vi "Teleop.vi"(10 "Match Info":T1={"Autonomous Elapsed Seconds"=0.0, "TeleOp Elapsed Seconds"=0.0, "Disabled Elapsed Seconds"=0.0, "Visited Autonomous"=FALSE, "Visited TeleOp"=FALSE, "Visited Disabled"=FALSE, "Autonomous Settings"={"Autonomous Style"=enum."Independent", "VI Refnum"=refnum}}, 11 "Call Context":T2) -> ()   [LabVIEW 2011]
doc: "This VI is called for each TeleOp packet received from the DS where the robot is not disabled. It is often used to read from the joysticks and update I/O or to update setpoints for timed control loops. It should complete and return within 20 milliseconds or it may miss DS packets."
uses:
  <vilib>/Rock Robotics/WPI/DriverStation/WPI_DriverStationDerivedRobotMode.ctl
  <vilib>/Rock Robotics/WPI/DriverStation/WPI_DriverStationMatch Info.ctl
  Robot Global Data.vi
panel:
  out "Target Angle":dbl
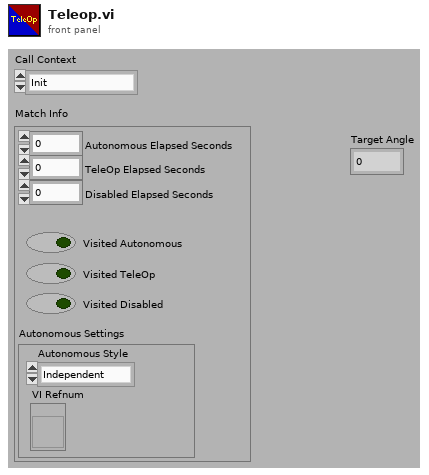
[diagram p1: front panel]
types:
  T1 = typedef "WPI_DriverStationMatch Info.ctl" = cluster{"Autonomous Elapsed Seconds":dbl, "TeleOp Elapsed Seconds":dbl, "Disabled Elapsed Seconds":dbl, "Visited Autonomous":bool, "Visited TeleOp":bool, "Visited Disabled":bool, "Autonomous Settings":cluster{"Autonomous Style":enum16{"Iterative", "Independent"}, "VI Refnum":refnum<vi>}}
  T2 = typedef "WPI_DriverStationDerivedRobotMode.ctl" = enum16{"Init", "Execute", "Stop"}
  T3 = typedef "WPI_JoystickDevRef.ctl" = cluster{"Device":T4}
  T4 = typedef "WPI_JoystickDeviceEnum.ctl" = enum16{"USB 1", "USB 2", "USB 3", "USB 4", "Kinect 1", "Kinect 2"}
  T5 = cluster{"Shooter Warmup":bool, "Shooter Allow Fire":bool}
  T6 = typedef "WPI_JoystickButtonState.ctl" = cluster{"Button 1":bool, "Button 2":bool, "Button 3":bool, "Button 4":bool, "Button 5":bool, "Button 6":bool, "Button 7":bool, "Button 8":bool, "Button 9":bool, "Button 10":bool, "Button 11":bool, "Button 12":bool}
  T7 = cluster{"axis 1 (x)":dbl, "axis 2 (y)":dbl, "axis 3 (throttle)":dbl, "axis 4":dbl, "axis 5":dbl, "axis 6":dbl}
  T8 = typedef "WPI_RobotDriveDevRef.ctl" = cluster{"DevStatus":errorcluster, "Motors[]":T9[], "Square Inputs":bool, "Max Output":dbl, "Isochronous":bool}
  T9 = typedef "WPI_MotorControlDeviceRef.ctl" = cluster{"DeviceStatus":errorcluster, "Type":enum16{"PWM", "CAN"}, "PWM":cluster{"Digital Module":T10, "PWM Channel":T11, "DeadBand":T12}, "CAN":cluster{"Device Number":u8, "Control Mode":T13, "Semaphore":T14, "Max Vout":dbl}, "Invert":bool, "TransformRef":T15, "InvTransformRef":T15}
  T10 = typedef "FPGA_TypedefDigitalModule.ctl" = enum16{"Digital Module 1", "Digital Module 2"}
  T11 = typedef "FPGA_DIOPWMChannel.ctl" = enum8{"PWM 1", "PWM 2", "PWM 3", "PWM 4", "PWM 5", "PWM 6", "PWM 7", "PWM 8", "PWM 9", "PWM 10", "Invalid"}
  T12 = typedef "WPI_PWMDeadband.ctl" = cluster{"Name":string, "maxPositivePwm":i32, "minPositivePwm":i32, "centerPwm":i32, "maxNegativePwm":i32, "minNegativePwm":i32, "angularRange":u16}
  T13 = typedef "WPI_CANJaguar_ControlMode.ctl" = enum8{"Percent VBus", "Current", "Speed", "Position", "Voltage"}
  T14 = typedef "Semaphore RefNum" = refnum<k1>
  T15 = typedef "WPI_PWMTransform_ConPane.ctl" = refnum<vi>
  T16 = typedef "WPI_GyroDevRef.ctl" = cluster{"DevStatus":errorcluster, "Analog Module":T17, "Analog Channel":T18, "Offset":dbl, "Gain (VoltsPerDegree/Second)":dbl}
  T17 = typedef "FPGA_TypedefAnalogModule.ctl" = enum16{"Analog Module 1", "Analog Module 2"}
  T18 = typedef "FPGA_AIChannel.ctl" = enum8{"AI 1", "AI 2", "AI 3", "AI 4", "AI 5", "AI 6", "AI 7", "AI 8", "Invalid"}
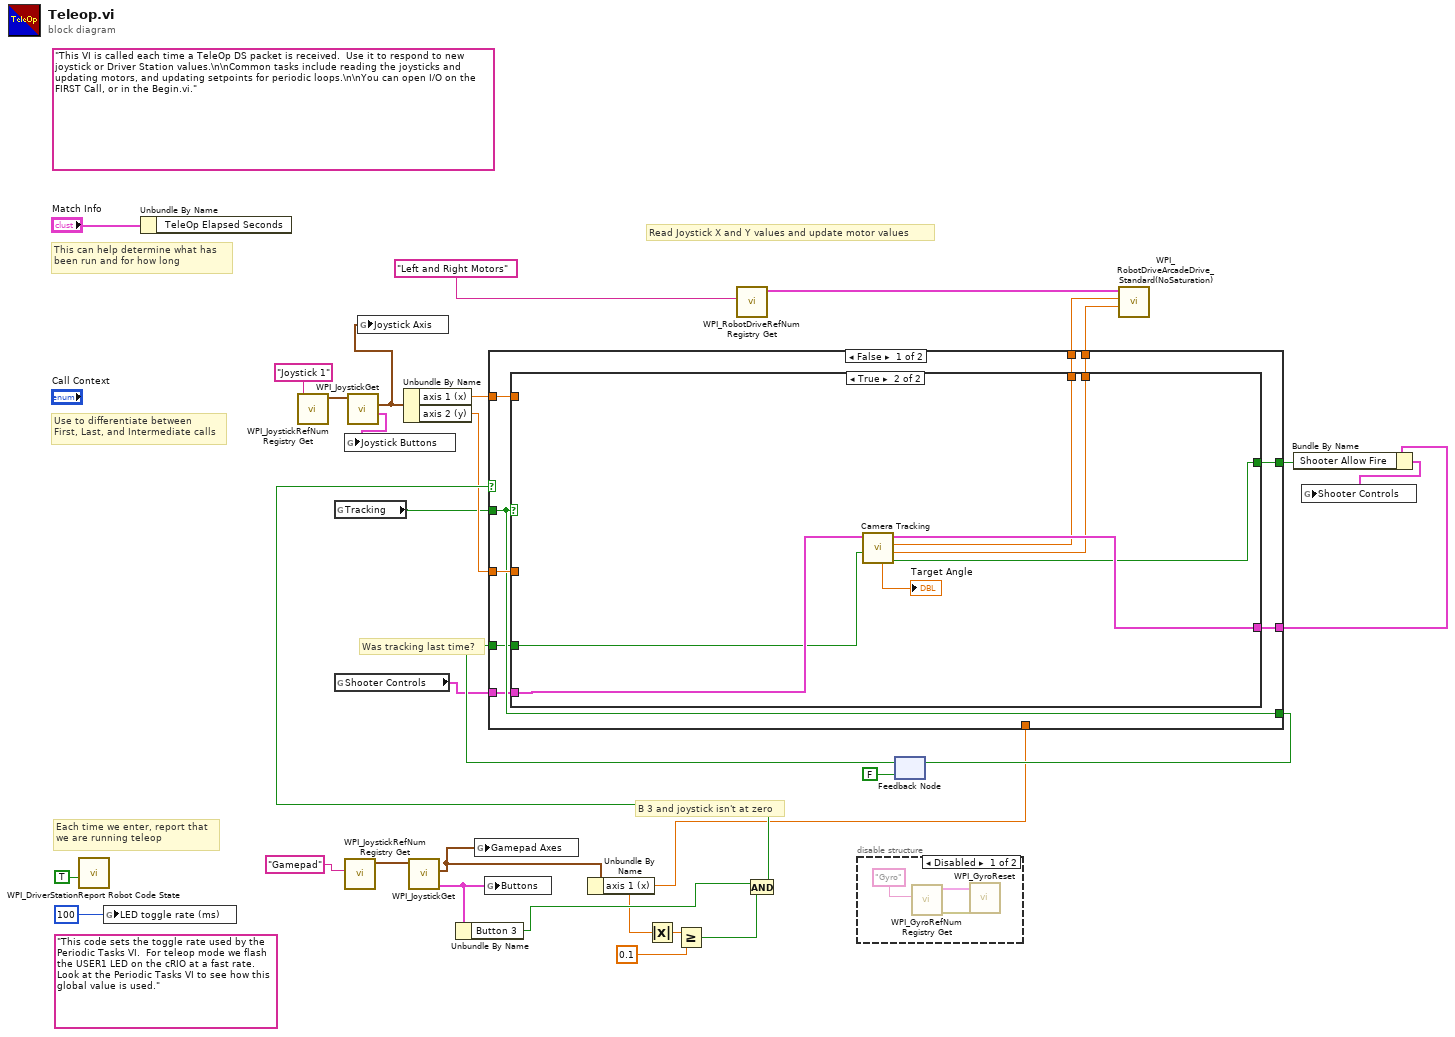
[diagram p0: block diagram]
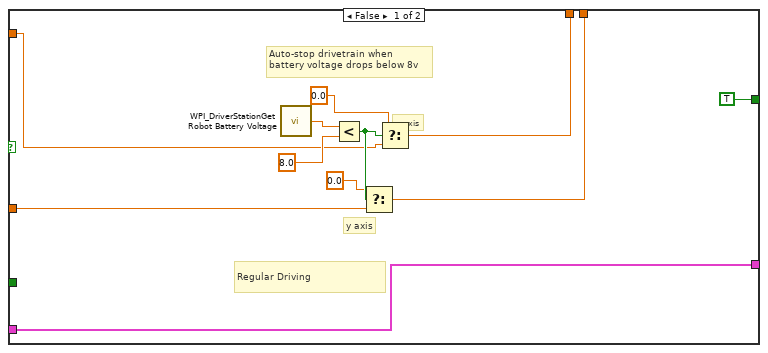
[diagram p3: hidden frame]
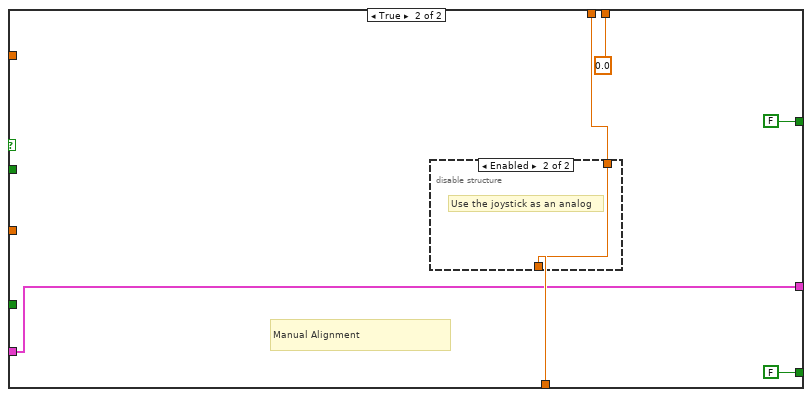
[diagram p4: hidden frame]
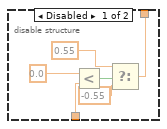
[diagram p5: hidden frame]
diagram:
  (unwired) "This code sets the toggle rate used by the Periodic Tasks VI.  For teleop mode we flash the USER1 LED on the cRIO at a fast rate.  Look at the Periodic Tasks VI to see how this global value is used."
  (unwired) "This VI is called each time a TeleOp DS packet is received.  Use it to respond to new joystick or Driver Station values.\n\nCommon tasks include reading the joysticks and updating motors, and updating setpoints for periodic loops.\n\nYou can open I/O on the FIRST Call, or in the Begin.vi."
  # "Was tracking last time?"
  # "B 3 and joystick isn't at zero"
  # "Each time we enter, report that\nwe are running teleop"
  # "Use to differentiate between\nFirst, Last, and Intermediate calls"
  # "This can help determine what has\nbeen run and for how long"
  # "Read Joystick X and Y values and update motor values"
  n1 = call <vilib>:"WPI_DriverStationReport Robot Code State.vi"("TeleOp"=TRUE ("Autonomous")) -> ()  [unwired: 10 in, 1 out]
  n2 = global write "Robot Global Data.vi" "LED toggle rate (ms)"(u32 100 ("LED ms toggle rate")) -> ()
  n3 = Unbundle By Name("Match Info") -> ()  [unwired: 1 out]
  n4 = call <vilib>:"WPI_JoystickRefNum Registry Get.vi"("refnum name"="Joystick 1") -> ("JoystickDevRef"=w16:T3)  [unwired: 1 in, 9 out]
  n5 = global read "Robot Global Data.vi" "Tracking"() -> (w4:bool)
  n6 = global read "Robot Global Data.vi" "Shooter Controls"() -> (w3:T5)
  n7 = call <vilib>:"WPI_JoystickRefNum Registry Get.vi"("refnum name"="Gamepad") -> ("JoystickDevRef"=w26:T3)  [unwired: 1 in, 9 out]
  n8 = call <vilib>:"WPI_JoystickGet.vi"("JoystickDevRef"=w16) -> ("Buttons"=w11:T6, "Axes"=w12:T7)  [unwired: 1 in, 4 out]
  n9 = global write "Robot Global Data.vi" "Joystick Buttons"(w11) -> ()
  n10 = global write "Robot Global Data.vi" "Joystick Axis"(w12) -> ()
  n11 = Unbundle By Name(w12) -> ("axis 1 (x)"=w13:dbl, "axis 2 (y)"=w14:dbl)
  n12 = call <vilib>:"WPI_JoystickGet.vi"("JoystickDevRef"=w26) -> ("Buttons"=w19:T6, "Axes"=w22:T7)  [unwired: 4 in, 1 out]
  n13 = Unbundle By Name(w19) -> ("Button 3"=w18:bool)
  n14 = global write "Robot Global Data.vi" "Gamepad Axes"(w22) -> ()
  n15 = global write "Robot Global Data.vi" "Buttons"(w19) -> ()
  n16 = Unbundle By Name(w22) -> ("axis 1 (x)"=w8:dbl)
  n17 = Absolute Value(x=w8) -> (abs(x)=w7:dbl)
  n18 = Greater Or Equal?(x=w7, y=0.1) -> (x >= y?=w20:bool)
  n19 = call <vilib>:"WPI_RobotDriveRefNum Registry Get.vi"("refnum name"="Left and Right Motors") -> ("RobotDriveDevRef"=w29:T8)  [unwired: 1 in, 9 out]
  n20 = And(x=w18, y=w20) -> (x .and. y?=w17:bool)
  n21 = disable-structure shown="Disabled" {
    frame Disabled {
      n22 = call <vilib>:"WPI_GyroRefNum Registry Get.vi"("refnum name"="Gyro") -> ("error out"=w34:errorcluster, "GyroDevRef"=w33:T16)  [unwired: 9 in]
      n23 = call <vilib>:"WPI_GyroReset.vi"("error in (no error)"=w34, "GyroDevRef"=w33) -> ()  [unwired: 8 in, 2 out]
    }
    frame Enabled {
    }
  }
  n24 = feedback #1(FALSE ("Button 3")) -> (w9:bool)
  n25 = case shown="False" w17 {
    tunnel: [w43 w65] -> w24
    tunnel: [w42 0.0 ("axis 2 (y)")] -> w23
    tunnel: w8 -> [_ w66]
    tunnel: w14 -> [w41 _]
    tunnel: w13 -> [w40 _]
    tunnel: w4 -> [w39 _]
    tunnel: [w39 FALSE ("Button 3")] -> w10
    tunnel: w9 -> [w38 _]
    tunnel: [w37 FALSE] -> w5
    tunnel: w3 -> [w36 w62]
    tunnel: [w35 w62] -> w2
    frame False {
      n26 = case shown="True" w39 {
        tunnel: [w50 w58] -> w43
        tunnel: [w49 w57] -> w42
        tunnel: w41 -> [w47 _]
        tunnel: w40 -> [w46 _]
        tunnel: w38 -> [_ w59]
        tunnel: [TRUE w56] -> w37
        tunnel: w36 -> [w44 w61]
        tunnel: [w44 w60] -> w35
        frame False {
          # "Auto-stop drivetrain when \nbattery voltage drops below 8v"
          # "Regular Driving"
          # "x axis"
          # "y axis"
          n27 = call <vilib>:"WPI_DriverStationGet Robot Battery Voltage.vi"() -> ("robot battery voltage"=w54:dbl)  [unwired: 14 in, 1 out]
          n28 = Less?(x=w54, y=8.0) -> (x < y?=w52:bool)
          n29 = Select(t=0.0, s=w52, f=w47) -> (s? t:f=w49:dbl)
          n30 = Select(t=0.0, s=w52, f=w46) -> (s? t:f=w50:dbl)
        }
        frame True {
          n31 = call "Camera Tracking.vi"("Was Tracking"=w59, "Shooter Controls"=w61) -> ("Aligned"=w56:bool, "Drive Y"=w57:dbl, "Drive X"=w58:dbl, "Shooter Controls Out"=w60:T5, "Target Angle"=→"Target Angle":dbl)  [unwired: 5 in]
        }
      }
    }
    frame True {
      # "Manual Alignment"
      n32 = disable-structure shown="Enabled" {
        disable-tunnel: w66 -> [w73 w74]
        disable-tunnel: [w68 w74] -> w65
        frame Disabled {
          n33 = Less?(x=0.0, y=w73) -> (x < y?=w71:bool)
          n34 = Select(t=0.55, s=w71, f=-0.55) -> (s? t:f=w68:dbl)
        }
        frame Enabled {
          # "Use the joystick as an analog"
        }
      }
    }
  }
  n35 = feedback-in #1(w10) -> ()
  n36 = call <vilib>:"WPI_RobotDriveArcadeDrive_Standard(NoSaturation).vi"("Y axis value"=w23, "X axis value"=w24, "RobotDriveDevRef"=w29) -> ()  [unwired: 1 in, 8 out]
  n37 = Bundle By Name(cluster=w2, "Shooter Allow Fire"=w5) -> (w1:T5)
  n38 = global write "Robot Global Data.vi" "Shooter Controls"(w1) -> ()
